vi "Read_LED.vi"(0 "COM Bluegiga in":refnum<visa-resource-name>, 1 "Characteristic UUID":string, 3 "Handle table":string[][](array[string]), 4 "Service UUID":string, 5 "error in (no error)":errorcluster, 13 "Connection Status":T1={"MAC Address"="", "cnx handle"=0, "cnx flags"=0, "Address Type"=125, "Connection Interval (ms)"=125, "Timeout(ms)"=125, "Latency"=0, "bonding handle"=0} {"Address Type" items=["Public", "Random"]}) -> (8 "Registro Completo":u8[](array[numeric]), 9 "Intensidad (One Shot)":u8, 10 "Color (constant)":u32(colorbox), 11 "Color (One Shot)":u8, 14 "COM Bluegiga out":refnum<visa-resource-name>, 15 "Modo":u8, 16 "Color (Breathe)":u8, 17 "Intensidad (breathe)":u8, 18 "Delay (breathe)":u16, 19 "error out":errorcluster)   [LabVIEW 2020]
uses:
  <vilib>/BLE/type_def/connection_status_bundle.ctl
  <vilib>/BLE/type_def/address_type.ctl
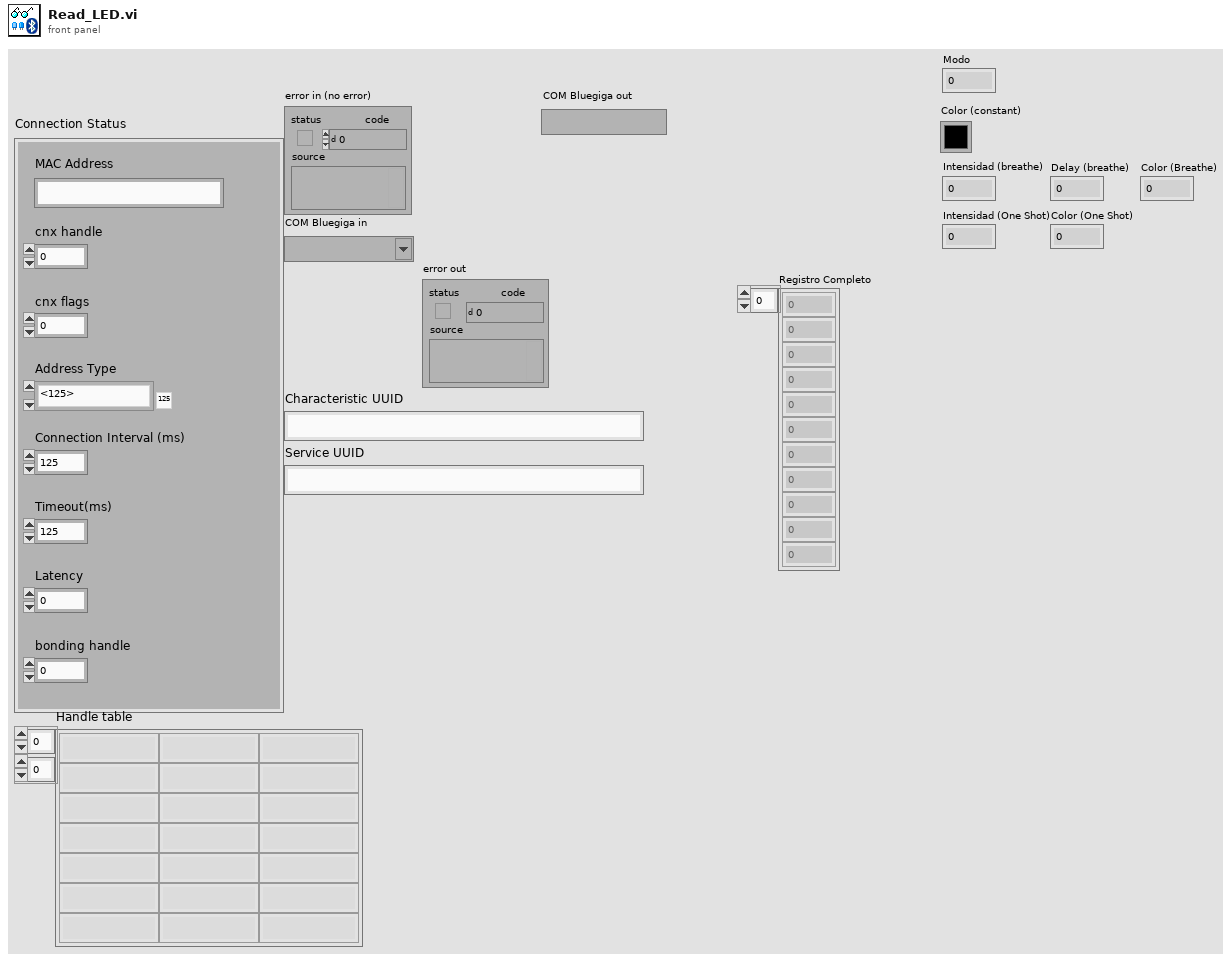
[diagram p1: front panel]
types:
  T1 = typedef "connection_status_bundle.ctl" = cluster{"MAC Address":string, "cnx handle":u8, "cnx flags":u8, "Address Type":T2, "Connection Interval (ms)":u16, "Timeout(ms)":u16, "Latency":u16, "bonding handle":u8}
  T2 = typedef "address_type.ctl" = u8
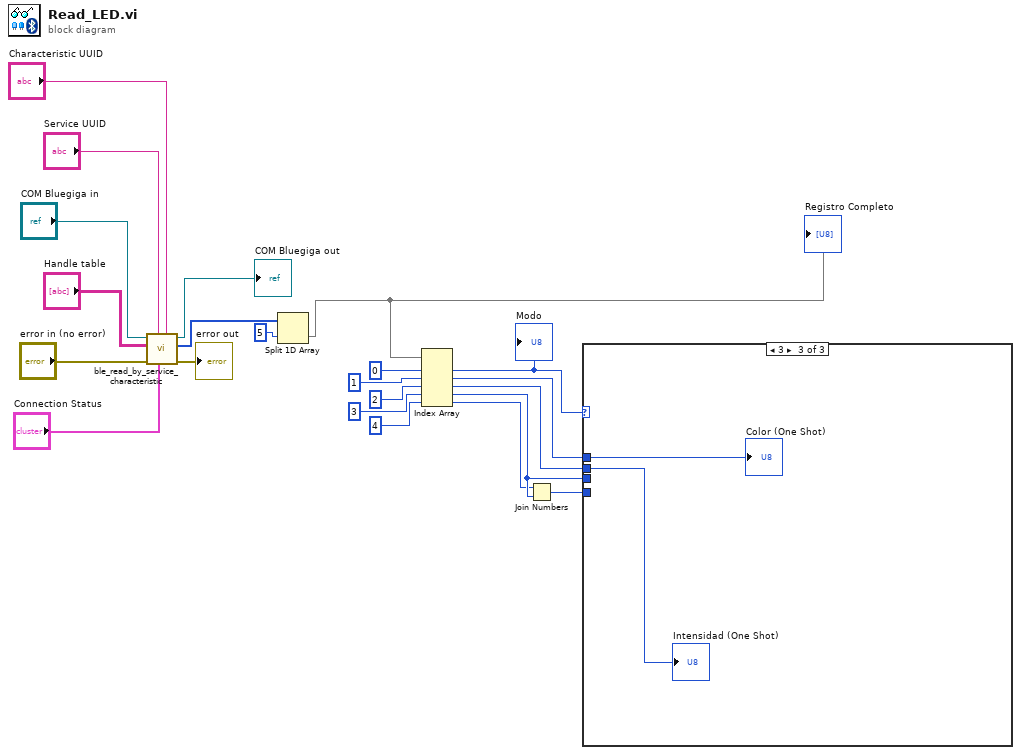
[diagram p0: block diagram]
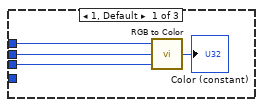
[diagram p2: hidden frame]
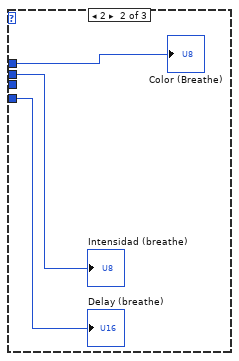
[diagram p3: hidden frame]
diagram:
  n1 = call <vilib>:"ble_read_by_service_characteristic.vi"("Characteristic UUID"="Characteristic UUID", "Connection Status"="Connection Status", "Service UUID"="Service UUID", "error in (no error)"="error in (no error)", "Handle table"="Handle table", "COM Bluegiga in"="COM Bluegiga in") -> ("error out"=→"error out":errorcluster, "characteristic value"=w21:u8[], "COM Bluegiga out"=→"COM Bluegiga out":refnum<visa-resource-name>)  [unwired: 3 in]
  n2 = Split 1D Array(array=w21, index=5) -> (second subarray=w12:u8[])  [unwired: 1 out]
  "Registro Completo" <- w12
  n3 = Index Array(array=w12, index #1=0 ("index"), index #2=1 ("index"), index #3=2 ("index"), index #4=3 ("index"), index #5=4 ("index")) -> (element #1=w10:u8, element #2=w9:u8, element #3=w8:u8, element #4=w2:u8, element #5=w1:u8)
  "Modo" <- w10
  n4 = Join Numbers(hi=w1, lo=w2) -> ((hi.lo)=w4:u16)
  n5 = case shown="3" w10 {
    tunnel: w9 -> [w25 w27 w30]
    tunnel: w8 -> [w24 w29 w31]
    tunnel: w2 -> [w23 _ _]
    tunnel: w4 -> [_ w28 _]
    frame 1, Default {
      n6 = call <vilib>:"RGB to Color.vi"("B"=w23, "G"=w24, "R"=w25) -> ("Color"=→"Color (constant)":u32)
    }
    frame 2 {
      "Intensidad (breathe)" <- w29
      "Delay (breathe)" <- w28
      "Color (Breathe)" <- w27
    }
    frame 3 {
      "Intensidad (One Shot)" <- w31
      "Color (One Shot)" <- w30
    }
  }
